vi "GraphSetupV2.vi"(8 "error in":errorcluster caption="entrée d'erreur (pas d'erreur)", 9 "PrefixeScan":string, 10 "PrefixeLog":string, 11 "InterfaceIn":refnum<class "Interface.lvclass">) -> (0 "error out":errorcluster caption="sortie d'erreur", 3 "InterfaceOut":refnum<class "Interface.lvclass">)   [LabVIEW 2010, in "Interface.lvclass"]
uses:
  Interface.lvclass
  GraphSetupStates.ctl
  Interface.lvclass/Interface.ctl
  <vilib>/Utility/error.llb/DialogType.ctl
panel:
  out "ScanlistItem":string
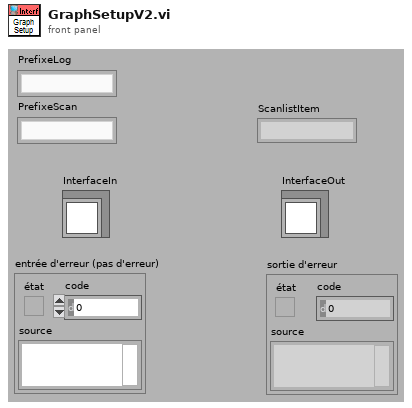
[diagram p1: front panel]
types:
  T1 = typedef "Interface.lvclass/GraphSetupStates.ctl" = enum16{"RdScnList", "UpdtGrphCurvs", "UpdtAllCurv", "SetGraphPar", "UpdtCrvPar", "GetNextItem", "UpdateGraph"}
  T2 = typedef "Interface.lvclass/CurveSetup.ctl" = cluster{"CurveName":string, "YParam":string, "XParam":string, "ZParam ":string, "GroupName":string, "LinWdth":u8, "PntCol":u32, "LinCol":u32, "LablFor":u8, "XScale":u32, "YScale":u32, "Interpol":u8, "DisplayName":string, "FillType":i16, "LineStyle":u8, "PntStyle":u8, "BarTyp":u8, "GraphIndex":i32, "Visible":bool, "XScaleName":string, "YScaleName":string, "XYGraph_Ref":refnum<vi>, "Data Only":bool, "DataQ Ref":refnum<queue>, "XParQ Ref":refnum<queue>, "XParamInd":i32}
  T3 = typedef "DialogType.ctl" = u16
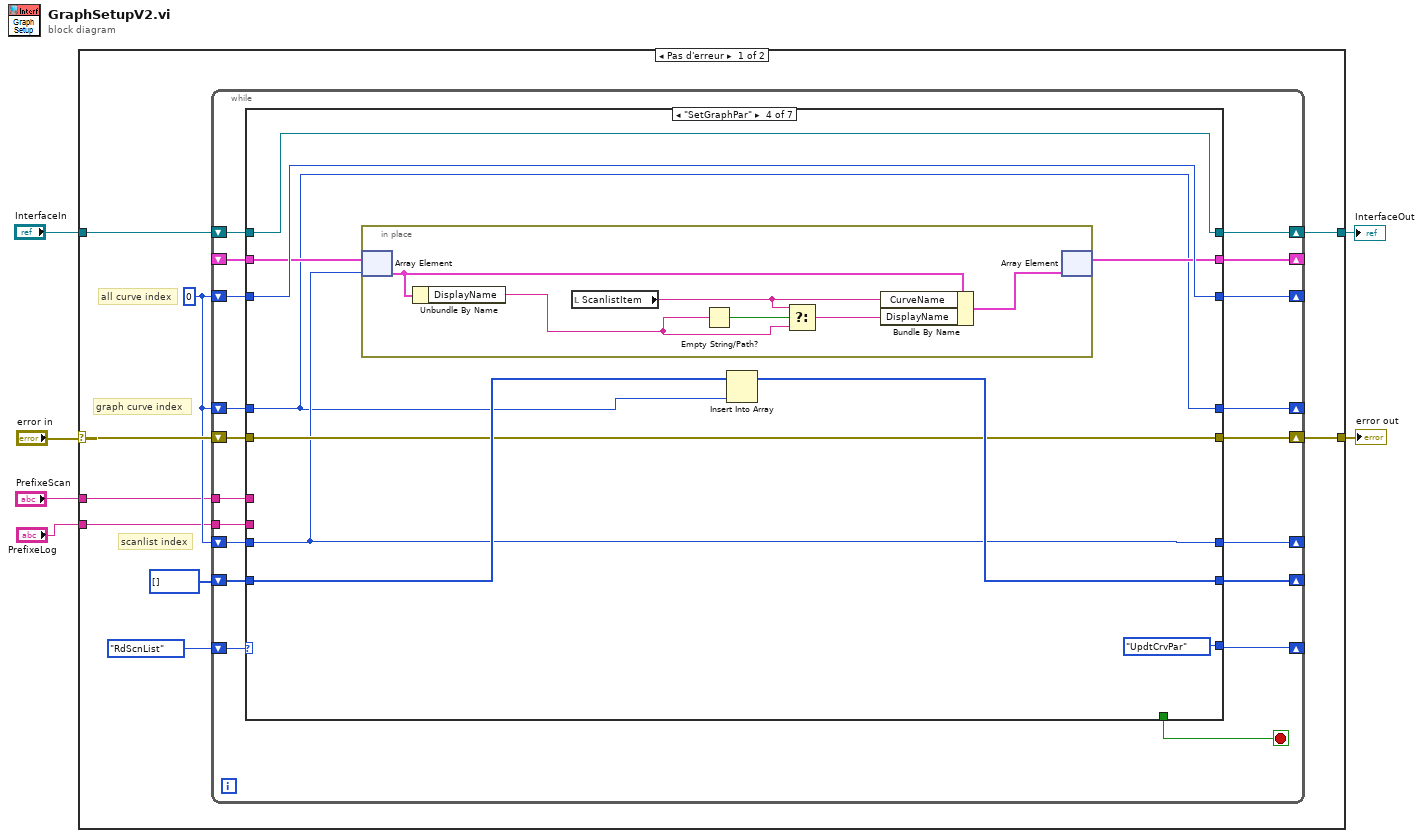
[diagram p0: block diagram]
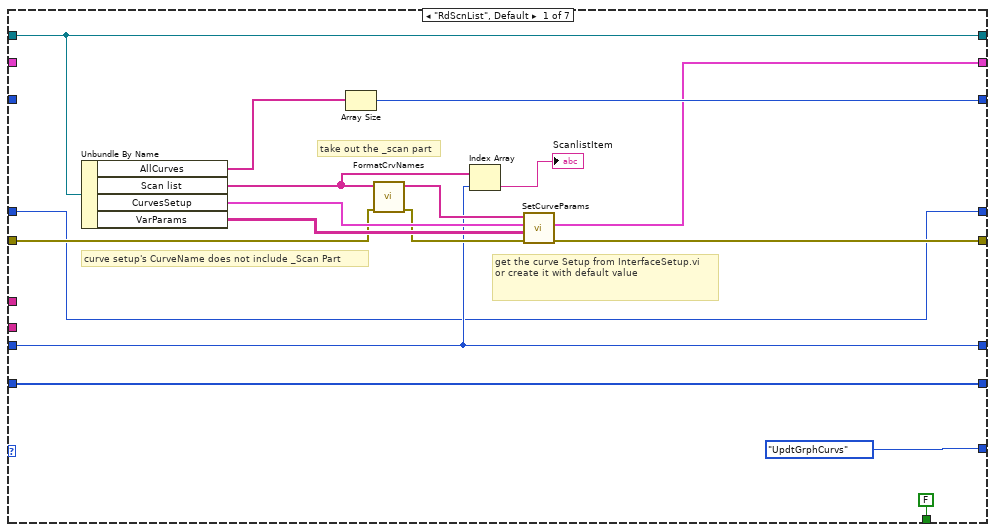
[diagram p2: hidden frame]
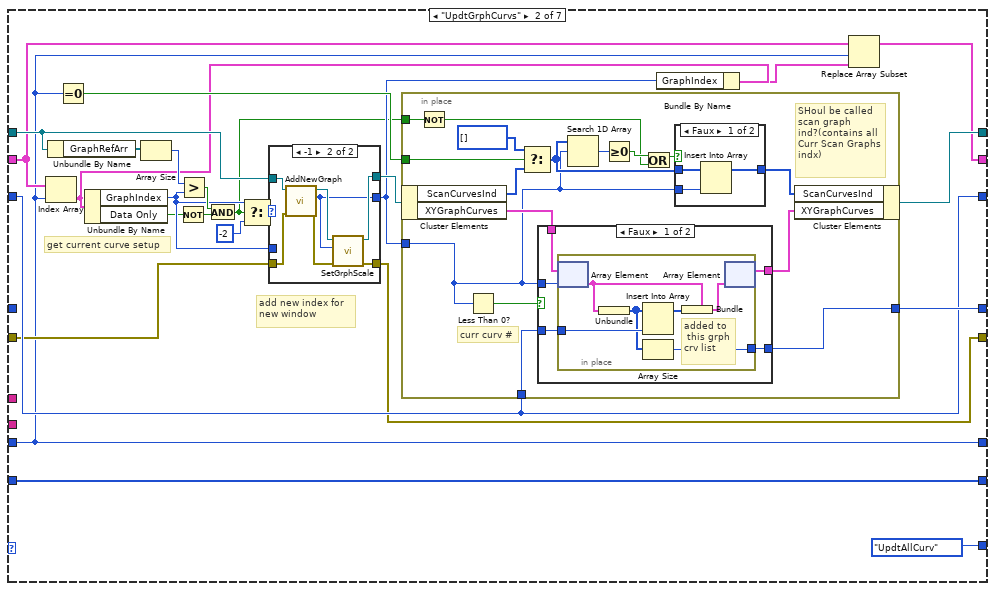
[diagram p3: hidden frame]
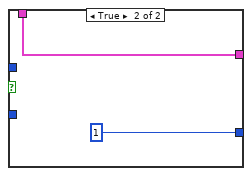
[diagram p4: hidden frame]
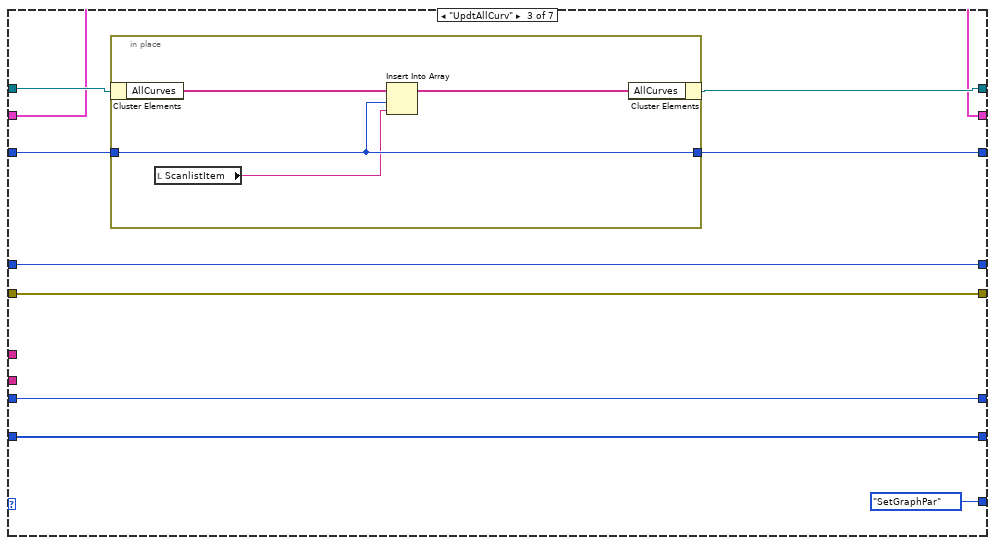
[diagram p7: hidden frame]
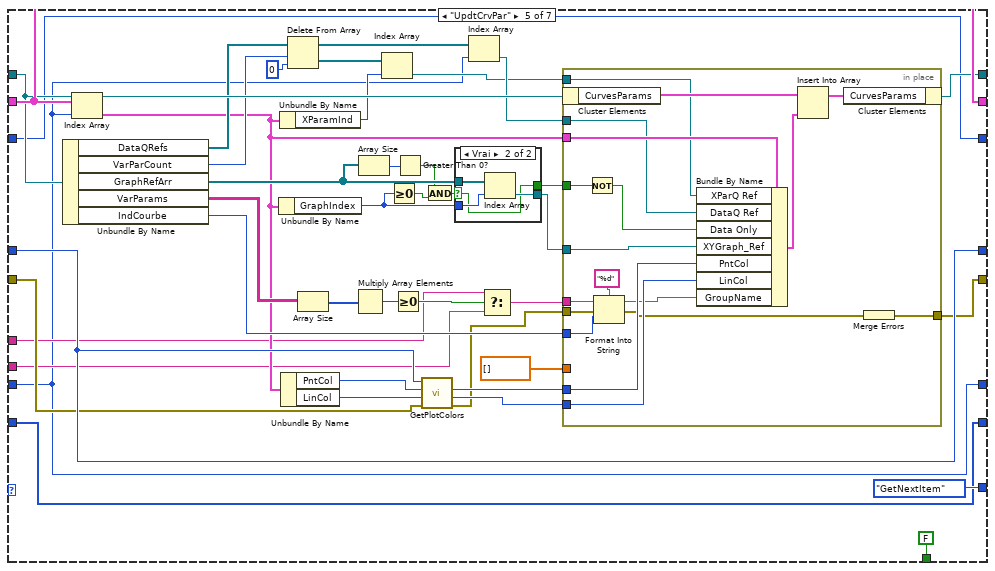
[diagram p8: hidden frame]
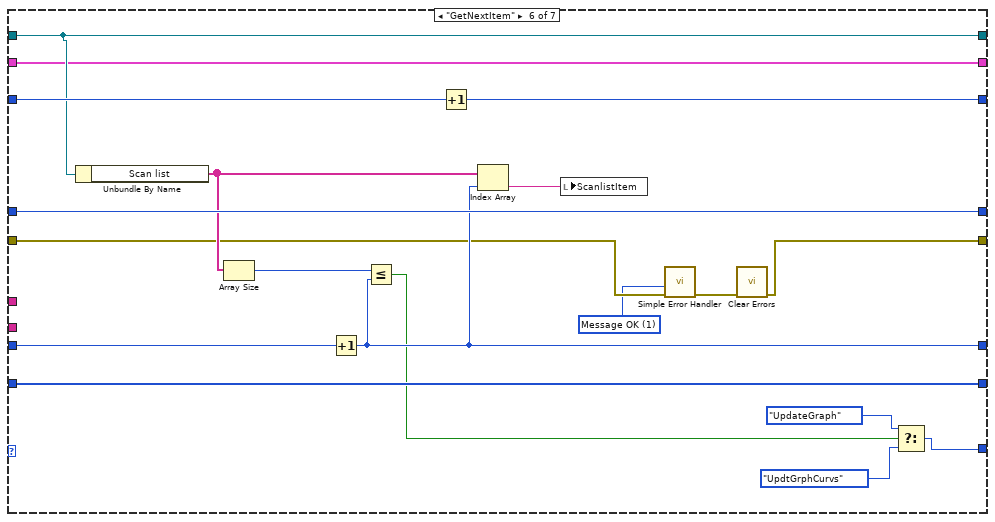
[diagram p10: hidden frame]
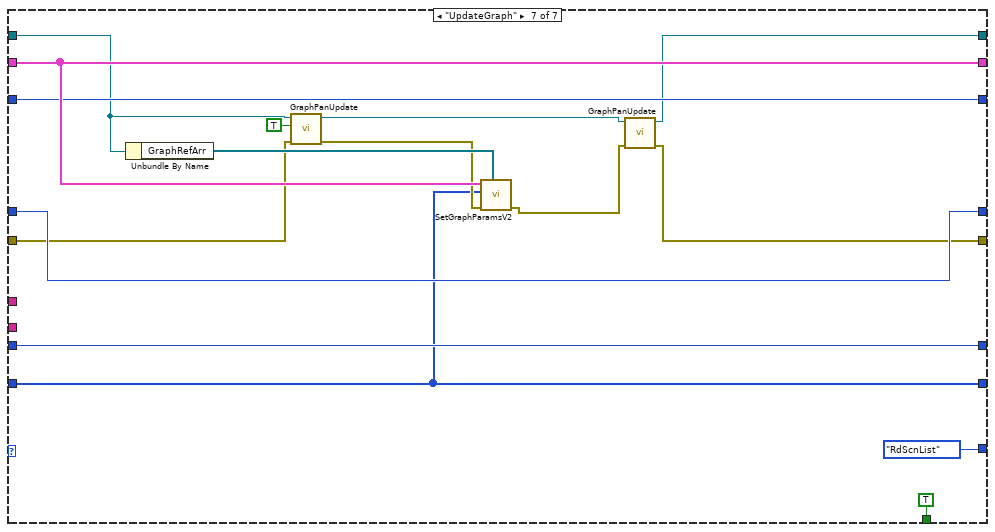
[diagram p11: hidden frame]
diagram:
  n1 = case shown="Pas d'erreur" "error in" {
    selector: "error in" -> [w15 w251]
    tunnel: [w14 w251] -> w5
    tunnel: "InterfaceIn" -> [w10 w250]
    tunnel: [w11 w250] -> w3
    tunnel: "PrefixeScan" -> [w9 _]
    tunnel: "PrefixeLog" -> [w8 _]
    frame No Error {
      w12 = 0
      # "scanlist index"
      # "graph curve index"
      # "all curve index"
      n2 = while {
        shift-right: [w25] -> w14
        shift-left: w15 -> [w26]
        shift-right: [w28] -> _
        shift-left: GraphSetupStates."RdScnList" ("Énum") -> [w20]
        shift-right: [w29] -> w11
        shift-left: w10 -> [w33]
        shift-right: [w32] -> _
        shift-left: w12 -> [w31]
        shift-right: [w30] -> _
        shift-left: w12 -> [w27]
        shift-right: [w24] -> _
        shift-left: _ -> [w23]
        shift-right: [w21] -> _
        shift-left: w12 -> [w22]
        tunnel: w9 -> [w19]
        tunnel: w8 -> [w18]
        shift-right: [w16] -> _
        shift-left: i32[] [] ("CuurGrphCrvInd") -> [w17]
        stop <- w34 stop-if-true
        n3 = case shown="\"SetGraphPar\"" w20 {
          tunnel: [FALSE _ _ _ FALSE _ TRUE] -> w34
          tunnel: w33 -> [w37 w69 w129 w141 w186 w230 w242]
          tunnel: [w47 w74 w125 w143 w151 w232 w243] -> w32
          tunnel: w31 -> [_ w74 w126 w143 w151 w233 w243]
          tunnel: [w38 w75 w121 w134 w181 w231 w247] -> w30
          tunnel: [w37 w70 w128 w141 w188 w230 w235] -> w29
          tunnel: [GraphSetupStates."UpdtGrphCurvs" ("Énum") GraphSetupStates."UpdtAllCurv" ("Énum") GraphSetupStates."SetGraphPar" ("Énum") GraphSetupStates."UpdtCrvPar" ("Énum") GraphSetupStates."GetNextItem" ("Énum") w215 GraphSetupStates."RdScnList" ("Énum")] -> w28
          tunnel: w27 -> [w38 _ w121 w134 w181 w231 w247]
          tunnel: w26 -> [w43 w73 w122 w138 w177 w222 w239]
          tunnel: [w41 w71 w122 w138 w176 w220 w236] -> w25
          tunnel: [w40 w60 w124 w136 w190 w229 w248] -> w24
          tunnel: w23 -> [_ w61 w124 w137 w190 w229 w248]
          tunnel: w22 -> [w39 w58 w123 w135 w152 w228 w246]
          tunnel: [w39 w58 w123 w135 w152 w225 w246] -> w21
          tunnel: w19 -> [_ _ _ _ w155 _ _]
          tunnel: w18 -> [_ _ _ _ w154 _ _]
          tunnel: w17 -> [w35 w52 w120 w140 w150 w219 w234]
          tunnel: [w35 w52 w120 w139 w150 w219 w234] -> w16
          frame "RdScnList", Default {
            # "take out the _scan part"
            # "get the curve Setup from InterfaceSetup.vi\nor create it with default value"
            # "curve setup's CurveName does not include _Scan Part"
            n4 = Unbundle By Name(w37) -> ("AllCurves"=w46:string[], "Scan list"=w45:string[], "CurvesSetup"=w49:T2[], "VarParams"=w50:string[][])
            n5 = Array Size(array=w46) -> (size(s)=w47:i32)
            n6 = call "FormatCrvNames.vi"("entrée d'erreur"=w43, "CurveNamesIn"=w45) -> ("sortie d'erreur"=w42:errorcluster, "CurveNames"=w51:string[])  [unwired: 8 in]
            n7 = Index Array(array=w45, index=w39) -> (element=→"ScanlistItem":string)
            n8 = call "SetCurveParams.vi"("error in (no error)"=w42, "VarParams"=w50, "CurveSetupsIn"=w49, "CurveNames"=w51) -> ("error out"=w41:errorcluster, "CurveSetupsOut"=w40:T2[])  [unwired: 6 in]
          }
          frame "UpdtGrphCurvs" {
            # "add new index for new window"
            # "get current curve setup"
            n9 = Index Array(array=w61, index=w58) -> (element=w59:T2)
            n10 = Unbundle By Name(w69) -> ("GraphRefArr"=w67:refnum<vi>[])
            n11 = Equal To 0?(x=w58) -> (x = 0?=w62:bool)
            n12 = Unbundle By Name(w59) -> ("GraphIndex"=w65:i32, "Data Only"=w55:bool)
            n13 = Array Size(array=w67) -> (size(s)=w68:i32)
            n14 = Not(x=w55) -> (.not. x?=w54:bool)
            n15 = Greater?(x=w68, y=w65) -> (0:w66:bool)
            n16 = And(x=w66, y=w54) -> (x .and. y?=w53:bool)
            n17 = Select(t=w65, s=w53, f=-2 ("cas faux")) -> (s? t:f=w63:i32)
            n18 = case shown="-1" w63 {
              selector: w63 -> [w110 _]
              tunnel: w65 -> [_ _]
              tunnel: [w110 w113] -> w56
              tunnel: w69 -> [w112 w119]
              tunnel: w73 -> [w111 w118]
              tunnel: [w112 w116] -> w72
              tunnel: [w111 w114] -> w71
              frame Default {
              }
              frame -1 {
                n19 = call "AddNewGraph.vi"("error in (no error)"=w118, "Interface en entrée"=w119) -> ("error out"=w115:errorcluster, "NewGraphInd"=w113:i32, "Interface en sortie"=w117:refnum<class "Interface.lvclass">)  [unwired: 7 in]
                n20 = call "SetGrphScale.vi"("error in (no error)"=w115, "GraphIndex"=w113, "Interface en entrée"=w117) -> ("error out"=w114:errorcluster, "Interface en sortie"=w116:refnum<class "Interface.lvclass">)  [unwired: 7 in]
              }
            }
            n21 = in-place {
              in-place-border: [w92] -> w75
              in-place-border: w74 -> [w83]
              in-place-border: w62 -> [w91]
              in-place-border: w56 -> [w82]
              in-place-border: w53 -> [w79]
              # "curr curv #"
              # "SHoul be called\nscan graph ind?(contains all Curr Scan Graphs indx)"
              n22 = in-place-cluster #1(w72) -> ("ScanCurvesInd"=w87:i32[], "XYGraphCurves"=w89:cluster{"Tableau":i32[]}[])
              n23 = Not(x=w79) -> (.not. x?=w77:bool)
              n24 = Less Than 0?(x=w82) -> (x < 0?=w81:bool)
              n25 = Select(t=i32[] [] ("cas vrai"), s=w91, f=w87) -> (s? t:f=w85:i32[])
              n26 = case shown="Faux" w81 {
                tunnel: [w97 1] -> w92
                tunnel: w83 -> [w96 _]
                tunnel: w89 -> [w95 w105]
                tunnel: [w94 w105] -> w88
                tunnel: w82 -> [w93 _]
                frame False {
                  n27 = in-place {
                    in-place-border: [w103] -> w97
                    in-place-border: w96 -> [w102]
                    # "added to\n this grph\ncrv list"
                    n28 = in-place-array #2(w95, w93) -> (w99:cluster{"Tableau":i32[]})
                    n29 = Unbundle(w99) -> ("Tableau"=w101:i32[])
                    n30 = Insert Into Array(array=w101, new element=w102) -> (w100:i32[])  [unwired: 1 in]
                    n31 = Array Size(array=w101) -> (size(s)=w103:i32)
                    n32 = Bundle(cluster=w99, "Tableau"=w100) -> (w98:cluster{"Tableau":i32[]})
                    n33 = in-place-array #2(w98) -> (w94:cluster{"Tableau":i32[]}[])  [unwired: 1 out]
                  }
                }
                frame True {
                }
              }
              n34 = Search 1D Array(1D array=w85, element=w82) -> (index of element=w84:i32)  [unwired: 1 in]
              n35 = Greater Or Equal To 0?(x=w84) -> (x >= 0?=w78:bool)
              n36 = Or(x=w78, y=w77) -> (x .or. y?=w80:bool)
              n37 = case shown="Faux" w80 {
                tunnel: [w108 w109] -> w86
                tunnel: w85 -> [w107 w109]
                tunnel: w82 -> [w106 _]
                frame False {
                  n38 = Insert Into Array(array=w107, new element=w106) -> (w108:i32[])  [unwired: 1 in]
                }
                frame True {
                  # "already in"
                }
              }
              n39 = in-place-cluster #1("ScanCurvesInd"=w86, "XYGraphCurves"=w88) -> (w70:refnum<class "Interface.lvclass">)
            }
            n40 = Bundle By Name(cluster=w59, "GraphIndex"=w56) -> (w57:T2)
            n41 = Replace Array Subset(array=w61, new element=w57, index=w58) -> (w60:T2[])
          }
          frame "UpdtAllCurv" {
            n42 = in-place {
              in-place-border: w126 -> [w131]
              in-place-border: [w131] -> w125
              n43 = in-place-cluster #3(w129) -> ("AllCurves"=w133:string[])
              n44 = local read "ScanlistItem"() -> (w130:string)
              n45 = Insert Into Array(array=w133, index=w131, new element=w130) -> (w132:string[])
              n46 = in-place-cluster #3("AllCurves"=w132) -> (w128:refnum<class "Interface.lvclass">)
            }
          }
          frame "SetGraphPar" {
            n47 = in-place {
              n48 = in-place-array #4(w137, w135) -> (w149:T2)
              n49 = Unbundle By Name(w149) -> ("DisplayName"=w147:string)
              n50 = local read "ScanlistItem"() -> (w146:string)
              n51 = Empty String/Path?(string/path=w147) -> (empty?=w148:bool)
              n52 = Select(t=w146, s=w148, f=w147) -> (s? t:f=w145:string)
              n53 = Bundle By Name(cluster=w149, "CurveName"=w146, "DisplayName"=w145) -> (w144:T2)
              n54 = in-place-array #4(w144) -> (w136:T2[])  [unwired: 1 out]
            }
            n55 = Insert Into Array(array=w140, new element=w134) -> (w139:i32[])  [unwired: 1 in]
          }
          frame "UpdtCrvPar" {
            n56 = Unbundle By Name(w186) -> ("DataQRefs"=w167:refnum<queue>[], "VarParCount"=w166:i32, "GraphRefArr"=w174:refnum<vi>[], "VarParams"=w163:string[][], "IndCourbe"=w178:i64)
            n57 = Index Array(array=w190, index=w152) -> (element=w160:T2)
            n58 = Unbundle By Name(w160) -> ("GraphIndex"=w175:i32)
            n59 = Unbundle By Name(w160) -> ("XParamInd"=w159:i32)
            n60 = Unbundle By Name(w160) -> ("PntCol"=w183:u32, "LinCol"=w182:u32)
            n61 = Delete From Array(array=w167, length=w166, index=0 ("indice")) -> (deleted portion=w161:refnum<queue>[], array with subset deleted=w165:refnum<queue>[])
            n62 = Array Size(array=w163) -> (size(s)=w185:i32[])
            n63 = Multiply Array Elements(1:w185) -> (0:w184:i32)
            n64 = Array Size(array=w174) -> (size(s)=w170:i32)
            n65 = Index Array(array=w161, index=w159) -> (element=w158:refnum<queue>)
            n66 = Greater Or Equal To 0?(x=w175) -> (x >= 0?=w172:bool)
            n67 = Greater Or Equal To 0?(x=w184) -> (x >= 0?=w157:bool)
            n68 = Greater Than 0?(x=w170) -> (x > 0?=w171:bool)
            n69 = call "GetPlotColors.vi"("ErrorIn(No Error)"=w177, "Color2In"=w182, "Color1In"=w183, "ColorIndex"=w181) -> ("sortie d'erreur"=w153:errorcluster, "Color2Out"=w179:u32, "Color1Out"=w180:u32)  [unwired: 4 in, 1 out]
            n70 = And(x=w171, y=w172) -> (x .and. y?=w173:bool)
            n71 = case shown="Vrai" w173 {
              selector: w173 -> [w192 w193]
              tunnel: [_ w196] -> w187
              tunnel: w174 -> [_ w195]
              tunnel: w175 -> [_ w194]
              tunnel: [w192 w193] -> w169
              frame False {
              }
              frame True {
                n72 = Index Array(array=w195, index=w194) -> (element=w196:refnum<vi>)
              }
            }
            n73 = Index Array(array=w165, index=w152) -> (element=w164:refnum<queue>)
            n74 = Select(t=w155, s=w157, f=w154) -> (s? t:f=w156:string)
            n75 = in-place {
              in-place-border: w187 -> [w212]
              in-place-border: w160 -> [w211]
              in-place-border: w180 -> [w209]
              in-place-border: w179 -> [w208]
              in-place-border: w156 -> [w206]
              in-place-border: w178 -> [w205]
              in-place-border: w153 -> [w199]
              in-place-border: [w198] -> w176
              in-place-border: w169 -> [w202]
              in-place-border: w164 -> [w200]
              in-place-border: dbl[] [] -> [_]
              in-place-border: w158 -> [w197]
              n76 = in-place-cluster #5(w186) -> ("CurvesParams"=w214:T2[])
              n77 = Not(x=w202) -> (.not. x?=w201:bool)
              n78 = Format Into String(format string="%d" ("chaîne de format"), initial string=w206, error in=w199, w205) -> (resulting string=w204:string, error out=w203:errorcluster)
              n79 = Bundle By Name(cluster=w211, "XParQ Ref"=w197, "DataQ Ref"=w200, "Data Only"=w201, "XYGraph_Ref"=w212, "PntCol"=w209, "LinCol"=w208, "GroupName"=w204) -> (w210:T2)
              n80 = Insert Into Array(array=w214, new element=w210) -> (w213:T2[])  [unwired: 1 in]
              n81 = in-place-cluster #5("CurvesParams"=w213) -> (w188:refnum<class "Interface.lvclass">)
              n82 = Merge Errors(w203) -> (w198:errorcluster)
            }
          }
          frame "GetNextItem" {
            w221 = T3 1 items=["pas de dialogue", "Message OK", "Message continuer ou arrêter", "Message OK + mises en garde", "Arrêter/Continuer + mises en garde"] ("type of dialog (OK msg:1)")
            n83 = Unbundle By Name(w230) -> ("Scan list"=w226:string[])
            n84 = Array Size(array=w226) -> (size(s)=w227:i32)
            n85 = Increment(x=w228) -> (x+1=w225:i32)
            n86 = Less Or Equal?(x=w227, y=w225) -> (x <= y?=w217:bool)
            n87 = Increment(x=w233) -> (x+1=w232:i32)
            n88 = Index Array(array=w226, index=w225) -> (element=w224:string)
            n89 = local write "ScanlistItem"(w224) -> ()
            n90 = call <vilib>:"Simple Error Handler.vi"("type of dialog (OK msg:1)"=w221, "error in (no error)"=w222) -> ("error out"=w223:errorcluster)  [unwired: 3 in, 4 out]
            n91 = call <vilib>:"Clear Errors.vi"("error in (no error)"=w223) -> ("error out"=w220:errorcluster)  [unwired: 6 in]
            n92 = Select(t=GraphSetupStates."UpdateGraph" ("Énum"), s=w217, f=GraphSetupStates."UpdtGrphCurvs" ("Énum")) -> (s? t:f=w215:T1)
          }
          frame "UpdateGraph" {
            n93 = Unbundle By Name(w242) -> ("GraphRefArr"=w249:refnum<vi>[])
            n94 = call "GraphPanUpdate.vi"("error in (no error)"=w239, "DeferUpdate"=TRUE, "Interface en entrée"=w242) -> ("error out"=w238:errorcluster, "Interface en sortie"=w240:refnum<class "Interface.lvclass">)  [unwired: 7 in]
            n95 = call "SetGraphParamsV2.vi"("GraphRefArr"=w249, "error in"=w238, "CuurGrphCrvInd"=w234, "CurveSetupsIn"=w248) -> ("error out"=w237:errorcluster)  [unwired: 7 in]
            n96 = call "GraphPanUpdate.vi"("error in (no error)"=w237, "Interface en entrée"=w240) -> ("error out"=w236:errorcluster, "Interface en sortie"=w235:refnum<class "Interface.lvclass">)  [unwired: 8 in]
          }
        }
      }
    }
    frame Error {
    }
  }
  "error out" <- w5
  "InterfaceOut" <- w3
